vi "Write OCP_Enable.vi"(8 "error in":errorcluster, 10 "OCP_Enable":bool, 11 "Acopian in":refnum<class "Acopian.lvclass">) -> (0 "error out":errorcluster, 3 "Acopian out":refnum<class "Acopian.lvclass">)   [LabVIEW 2019, in "Acopian.lvlib" / "Acopian.lvclass"]
uses:
  Library/Acopian.lvclass
  builds/Instruments/PowerSupply.lvlibp/Library/PowerSupply.lvclass
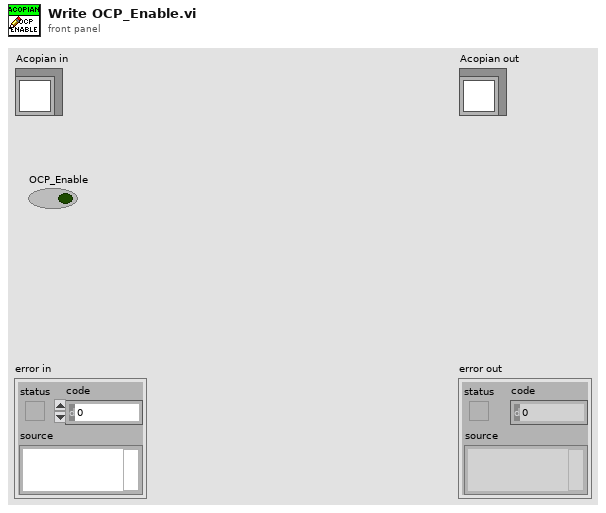
[diagram p1: front panel]
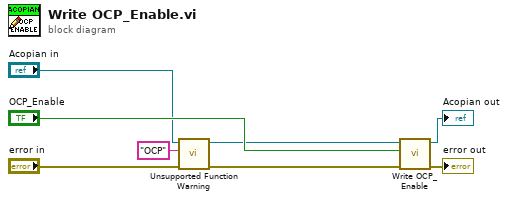
[diagram p0: block diagram]
diagram:
  n1 = call "Unsupported Function Warning.vi"("error in"="error in", "Unsupported Function"="OCP", "Acopian in"="Acopian in") -> ("error out"=w4:errorcluster, "Acopian out"=w3:refnum<class "Acopian.lvclass">)  [unwired: 7 in]
  n2 = call-parent "Write OCP_Enable.vi"("error in"=w4, "OCP_Enable"="OCP_Enable", "PowerSupply in"=w3) -> ("error out"=→"error out":errorcluster, "PowerSupply out"=→"Acopian out":refnum<class "Acopian.lvclass">)  [unwired: 7 in]
